vi "Fsweep_SR8XX.vi"() -> ()   [LabVIEW 2020]
panel:
  in  "data acq time (s)":dbl=2.0
  in  "coupled device":enum16{"SRS 8XXX", "Keithley 6221"}(ring)
  in  "base delay (ms)":dbl=2000.0
  in  "test mode":bool=TRUE
  out "done":u32=1
  out "delays (ms)":dbl[](array[numeric])=[4439.024390243903, 4404.322127575027, 4370.113606190229, 4336.391801174221, 4303.149787561701, 4270.38073891527, 4238.07792592359, 4206.234715019476, 4174.844567017659, 4143.901035771921, 4113.3977668513535, 4083.328496235426, 4053.687049027639, 4024.467338187478, 3995.663363280398, 3967.269209245602, 3939.2790451813516, 3911.687123147558, 3884.4877769854065, 3857.675421153779, 3831.244549582238, 3805.189734540312, 3779.505625522889, 3754.1869481514573, 3729.22850309098, 3704.6251649821834, 3680.3718813890364, 3656.4636717612, 3632.895626411248, 3609.6629055064286, 3586.760738074784, 3564.1844210253985, 3541.9293181825924, 3519.990859333863, 3498.364539291357, 3477.045916966707, 3456.0306144590327, 3435.314316155911, 3414.892767847138, 3394.7617758511064, 3374.9172061536083, 3355.354983558889, 3336.071090852786, 3317.0615679777693, 3298.3225112197197, 3279.8500724062824, 3261.640458116619, 3243.6899289024086, 3225.9947985199315, 3208.551433173076, 3191.3562507671204, 3174.4057201731257, 3157.696360502801, 3141.2247403936835, 3124.987477304485, 3108.981236820472, 3093.202731968722, 3077.648722543126, 3062.3160144389926, 3047.2014589971222, 3032.3019523572093, 3017.6144348204493, 3003.135890221209, 2988.863345307645, 2974.793869131124, 2960.924572444339, 2947.2526071079833, 2933.775165505871, 2920.4894799683775, 2907.3928222040795, 2894.482502739488, 2881.755870366748, 2869.2103115991986, 2856.843250134678, 2844.652146326465, 2832.634496661748, 2820.7878332475157, 2809.1097233037576, 2797.597768663886, 2786.24960528225, 2775.0629027486693, 2764.0353638098745, 2753.1647238977457, 2742.448750664277, 2731.8852435231465, 2721.4720331978187, 2711.206981276064, 2701.0879797708303, 2691.112950687351, 2681.279845596418, 2671.5866452137298, 2662.031358985212, 2652.6120246782516, 2643.3267079787383, 2634.173502093844, 2625.1505273604503, 2616.2559308591503, 2607.4878860337403, 2598.8445923161253, 2590.3242747565655, 2581.9251836591748, 2573.645594222615, 2565.483806185897, 2557.43814347922, 2549.506953879787, 2541.6886086725035, 2533.981502315518, 2526.3840521105117, 2518.8946978776826, 2511.5119016353547, 2504.2341472841445, 2497.0599402956186, 2489.9878074053895, 2483.0162963105668, 2476.143975371521, 2469.3694333178873, 2462.691278958754, 2456.108140896974, 2449.618667247538, 2443.2215253599597, 2436.9154015446074, 2430.6990008029316, 2424.571046561526, 2418.5302804099815, 2412.575461842458, 2406.705368002946, 2400.918793434141, 2395.2145498298987, 2389.5914657912076, 2384.048386585637, 2378.5841739102075, 2373.1977056576297, 2367.887875685877, 2362.6535935910315, 2357.493784483362, 2352.4073887665927, 2347.3933619203062, 2342.4506742854455, 2337.578310852868, 2332.7752710549103, 2328.04056855991, 2323.3732310696623, 2318.772300119751, 2314.2368308827204, 2309.7658919740543, 2305.358565260906, 2301.013945673557, 2296.731141019556, 2292.5092718005008, 2288.3474710314285, 2284.2448840627767, 2280.200668404874, 2276.2139935549317, 2272.284040826495, 2268.4100031813205, 2264.591085063646, 2260.82650223682, 2257.1154816222534, 2253.457261140662, 2249.851089555573, 2246.2962263190493, 2242.791941419618, 2239.3375152323556, 2235.932238371111, 2232.5754115428267, 2229.266345403937, 2226.0043604188077, 2222.7887867201857, 2219.6189639716436, 2216.4942412319715, 2213.4139768215036, 2210.3775381903474, 2207.384301788483, 2204.433652937716, 2201.524985705449, 2198.6577027802496, 2195.8312153491884, 2193.044942976925, 2190.298313486511, 2187.590762841889, 2184.9217350320673, 2182.290681956938, 2179.6970633147207, 2177.1403464910118, 2174.620006449405, 2172.1355256236757, 2169.686393811492, 2167.272108069646, 2164.892172610768, 2162.546098701516, 2160.23340456221, 2157.953615267897, 2155.706262650822, 2153.4908852042854, 2151.3070279878743, 2149.154242534032, 2147.032086755969, 2144.940124856872, 2142.8779272404145, 2140.845070422535]
  in  "back to initial frequencies":bool=TRUE
  out "delay sum (min)":dbl=9.36111299636738
  in  "index offset":u16=6
  out "freq profile":dbl[][](array[numeric])=[[40.99999999999999], [41.59176461968469], [42.19207034583551], [42.80104045466266], [43.41880000165687], [44.04547584727021], [44.68119668296755], [45.32609305765421], [45.980297404484844], [46.643944068059355], [47.31716933201128], [48.000111446994545], [48.692910659073924], [49.39570923852533], [50.108651509051946], [50.83188387742187], [51.56555486353358], [52.30981513091526], [53.06481751766459], [53.830717067834826], [54.607671063273884], [55.395839055923275], [56.19538290058288], [57.006466788148714], [57.829257279330584], [58.66392333885625], [59.51063637016918], [60.369570250627405], [61.24090136721011], [62.124808652739766], [63.02147362262691], [63.931080412145505], [64.85381581424615], [65.78986931791488], [66.73943314708613], [67.7027023001168], [68.67987458983036], [69.67115068413874], [70.67673414725078], [71.6968314814753], [72.73165216962732], [73.7814087180468], [74.84631670023795], [75.92659480113835], [77.02246486202736], [78.1341519260824], [79.26188428459274], [80.40589352384065], [81.56641457265877], [82.74368575067426], [83.93794881724882], [85.14944902112572], [86.37843515079277], [87.62515958557246], [88.8898783474497], [90.17285115364719], [91.47434146995997], [92.79461656485945], [94.13394756437879], [95.49260950778984], [96.87088140408437], [98.26904628926995], [99.6873912844931], [101.12620765500114], [102.5857908699552], [104.06644066310672], [105.56846109434923], [107.09216061215888], [108.6378521169361], [110.20585302526148], [111.79648533507905], [113.41007569182058], [115.04695545548357], [116.70746076867859], [118.39193262565769], [120.10071694233959], [121.8341646273455], [123.59263165406033], [125.37647913373338], [127.18607338963533], [129.02178603228427], [130.88399403575826], [132.7730798151091], [134.6894313048933], [136.63344203883705], [138.6055112306498], [140.6060438560061], [142.635450735709], [144.69414862005462], [146.78256027441444], [148.90111456605186], [151.05024655219347], [153.23039756937], [155.44201532404736], [157.68555398456584], [159.961474274406], [162.270243566801], [164.61233598071445], [166.9882324782033], [169.3984209631858], [171.8433963816362], [174.32366082322412], [176.83972362442165], [179.3921014730987], [181.98131851462713], [184.60790645951803], [187.2724046926108], [189.9753603838391], [192.71732860059532], [195.4988724217168], [198.32056305311735], [201.18297994508785], [204.08671091128878], [207.03235224946238], [210.02050886388508], [213.05179438958805], [216.1268313183711], [219.24625112663387], [222.4106944050545], [225.6208109901378], [228.87726009766294], [232.18071045805726], [235.53184045372393], [238.9313382583516], [242.37990197823493], [245.87823979563404], [249.42707011420487], [253.0271217065268], [256.67913386376034], [260.3838565474651], [264.14205054360764], [267.95448761879476], [271.8219506787592], [275.745233929134], [279.7251430385472], [283.7624953040704], [287.85811981905556], [292.01285764339394], [296.22756197623283], [300.50309833118376], [304.84034471406244], [309.2401918031909], [313.703543132304], [318.23131527609524], [322.82443803843955], [327.4838546433357], [332.2105219286013], [337.0054105423655], [341.86950514239686], [346.80380459830866], [351.80932219668233], [356.8870858491522], [362.0381383034912], [367.2635373577478], [372.5643560774688], [377.94168301606044], [383.3966224383289], [388.93029454724626], [394.54383571399273], [400.2383987113154], [406.0151529502572], [411.8752847203018], [417.81999743298553], [423.85051186902433], [429.9680664290081], [436.17391738771397], [442.46933915208774], [448.8556245229529], [455.33408496049384], [461.90605085357], [468.5728717929217], [475.33591684831447], [482.1965748496856], [489.1562546723486], [496.21638552631373], [503.37841724978426], [510.64382060688916], [518.0140875897129], [525.4907317246851], [533.0752883833896], [540.7693150978654], [548.5743918804517], [556.4921215482547], [564.5241300522919], [572.672066811395], [580.937605050924], [589.3224421463751], [597.828299971946], [606.4569252541323], [615.2100899304289], [624.0895915132061], [633.0972534588399], [642.2349255421697], [651.5044842363571], [660.9078330982352], [670.4469031592117], [680.1236533218164], [689.940070761976], [699.8981713370904], [710.0000000000003]]
  out "freqs":dbl[](array[numeric])=[710.0000000000003]
  out "delay (ms)":dbl=2140.845070422535
  out "elapsed time (min)":dbl
  in  "sweep mode":T1(ring)=enum."log"
  in  "size":u32=200
  in  "final":dbl=15000.0
  in  "initial":dbl=41.0
  in  "Device address":refnum<visa-resource-name>[](array[refnum])=["GPIB0::21::INSTR", "GPIB0::22::INSTR", "GPIB0::23::INSTR"]
  # "Test the frequency profile and the estimated measurement time (delay sum (min)) with the 'test mode on'\nTurn the test mode off for the real measurement."
  # "Start data acquistion  and frequency sweeps.\nStop the data acqusition when the sweep is done.\nVISA resource is opened and closed each time a command is executed."
  # "this delay time is added to the frequency dependent delay time"
  # "(1) For multiple lockins, the same freq profile is used but\nbut the starting frequency is offset to prevent crosstalking.\n(2) Ignored for a single lockin. \n* Check the context help"
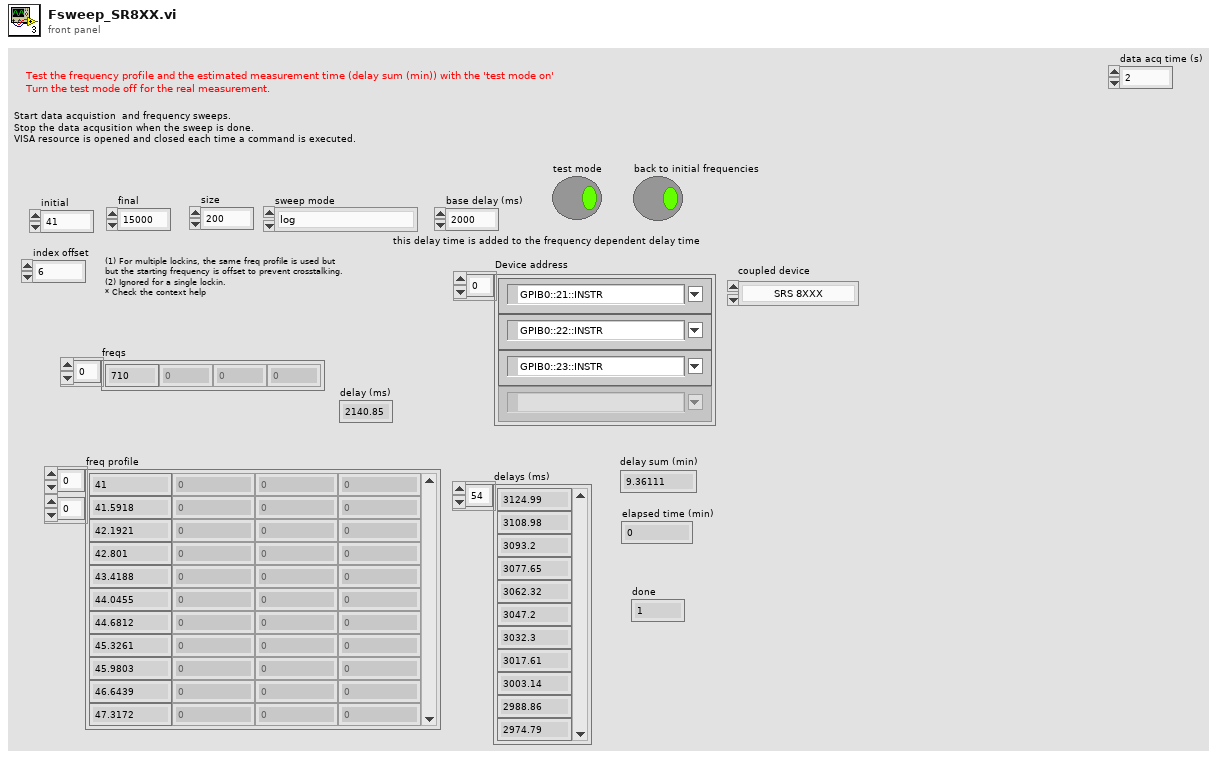
[diagram p1: front panel]
types:
  T1 = enum16{"linear", "inverse", "log", "inverse log"}
  T2 = enum32{"New", "Stop", "Trigger", "Delta Trigger", "Run", "Pause", "comments", "Started?"}
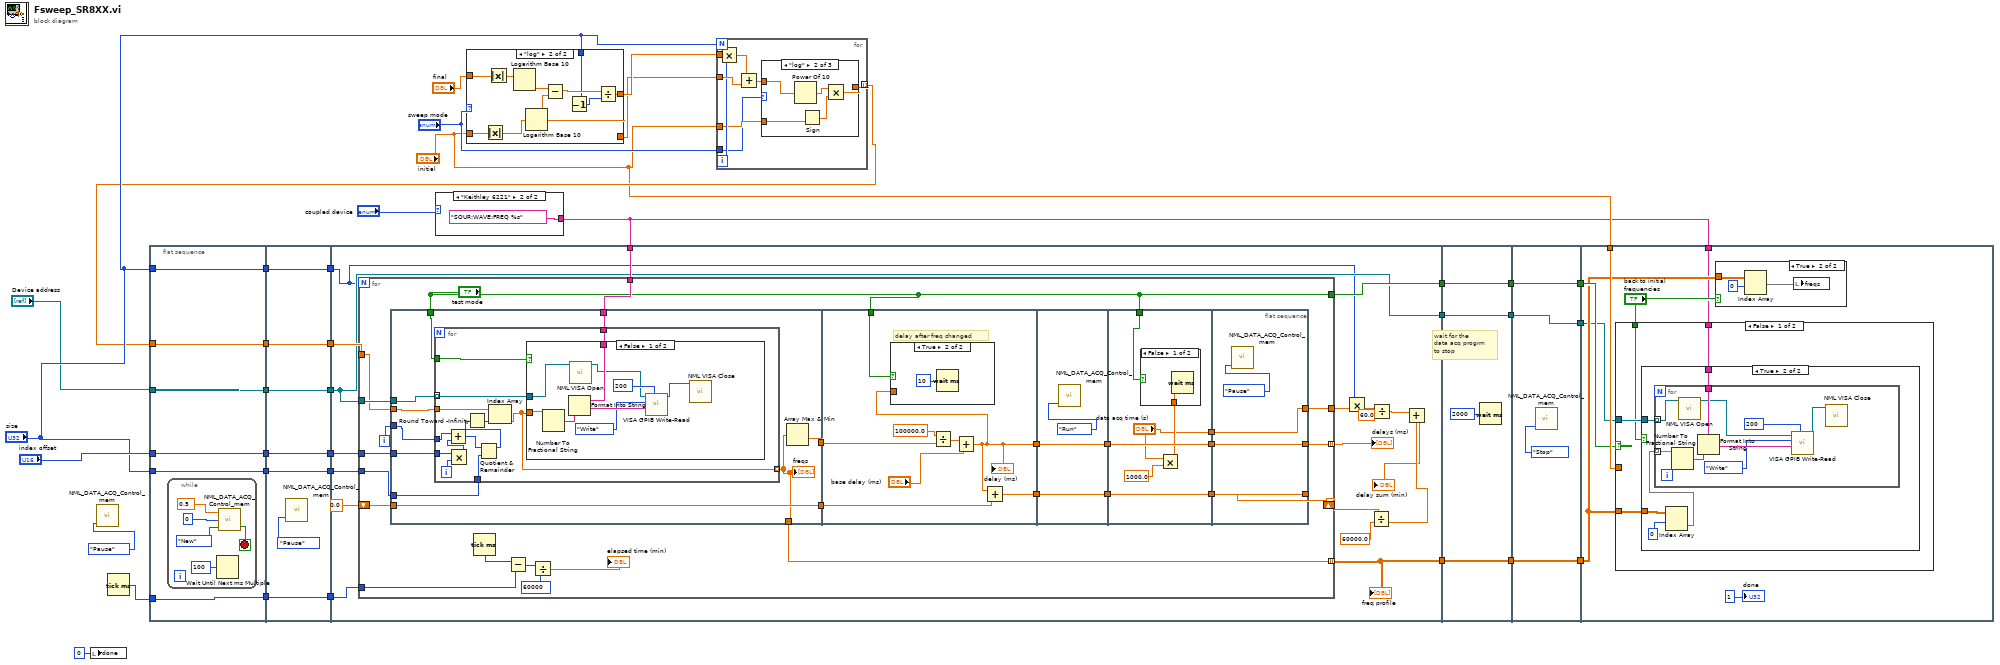
[diagram p0: block diagram]
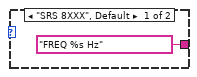
[diagram p2: hidden frame]
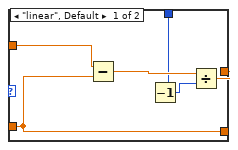
[diagram p3: hidden frame]
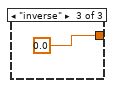
[diagram p5: hidden frame]
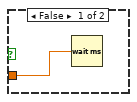
[diagram p7: hidden frame]
diagram:
  n1 = local write "done"(u32 0 ("done")) -> ()
  n2 = call "NML_DATA_ACQ_Control_mem.vi"("Enum"=T2."Pause") -> ()  [unwired: 4 in, 1 out]
  n3 = Tick Count (ms)() -> (millisecond timer value=w35:u32)
  n4 = flat-sequence {
    tunnel: "size" -> [w36]
    tunnel: "index offset" -> [w37]
    tunnel: "Device address" -> [w38]
    tunnel: "size" -> [w39]
    tunnel: w35 -> [w40]
    tunnel: w27 -> [w41]
    tunnel: [w41] -> w19
    tunnel: [w40] -> w17
    tunnel: [w39] -> w15
    tunnel: [w38] -> w13
    tunnel: [w37] -> w11
    tunnel: [w36] -> w9
    tunnel: w19 -> [w53]
    tunnel: [w53] -> w18
    tunnel: w17 -> [w52]
    tunnel: [w52] -> w16
    tunnel: w15 -> [w51]
    tunnel: [w51] -> w14
    tunnel: w13 -> [w50]
    tunnel: [w50] -> w12
    tunnel: w11 -> [w49]
    tunnel: [w49] -> w10
    tunnel: w9 -> [w48]
    tunnel: [w48] -> w8
    tunnel: [w71] -> w6
    tunnel: [w64] -> w4
    tunnel: w22 -> [w62]
    tunnel: [w61] -> w2
    tunnel: w18 -> [w72]
    tunnel: w16 -> [w70]
    tunnel: w14 -> [w59]
    tunnel: w12 -> [w61]
    tunnel: w10 -> [w69]
    tunnel: w8 -> [w68]
    tunnel: w6 -> [w158]
    tunnel: [w158] -> w5
    tunnel: w4 -> [w157]
    tunnel: [w157] -> w3
    tunnel: w2 -> [w156]
    tunnel: [w156] -> w1
    tunnel: w5 -> [w162]
    tunnel: [w162] -> w25
    tunnel: w3 -> [w161]
    tunnel: [w161] -> w24
    tunnel: [w160] -> w21
    tunnel: w1 -> [w160]
    tunnel: w25 -> [w168]
    tunnel: "initial" -> [w169]
    tunnel: w24 -> [w165]
    tunnel: w22 -> [w164]
    tunnel: w21 -> [w163]
    frame #0 {
      n5 = while {
        stop <- w43 stop-if-true
        n6 = Wait Until Next ms Multiple(millisecond multiple=u32 100) -> ()  [unwired: 1 out]
        n7 = call "NML_DATA_ACQ_Control_mem.vi"("Enum"=T2."New", "Trigger Column"=0, "Æ Trigger"=0.5) -> ("started"=w43:bool)  [unwired: 2 in]
      }
    }
    frame #1 {
      n8 = call "NML_DATA_ACQ_Control_mem.vi"("Enum"=T2."Pause") -> ()  [unwired: 4 in, 1 out]
    }
    frame #2 {
      n9 = for {
        N: w59 -> [_]
        tunnel: w72 -> [w83]
        tunnel: ["test mode"] -> w71
        tunnel: w70 -> [w97]
        tunnel: w61 -> [w93]
        tunnel: w69 -> [w91]
        tunnel: w68 -> [w90]
        tunnel: [w84] -> w64 mode=indexing
        tunnel: [w88] -> w63 mode=indexing
        shift-right: [w87] -> w65
        shift-left: 0.0 -> [w85]
        tunnel: w62 -> [w82]
        tunnel: [w73] -> w60
        i -> [w92]
        n10 = flat-sequence {
          tunnel: w83 -> [w106]
          tunnel: "test mode" -> [w108]
          tunnel: w93 -> [w107]
          tunnel: w92 -> [w105]
          tunnel: w91 -> [w104]
          tunnel: w90 -> [w103]
          tunnel: [w101] -> w89
          tunnel: [w100] -> w84
          tunnel: [w102] -> w86
          tunnel: w85 -> [w102]
          tunnel: w82 -> [w99]
          tunnel: w89 -> [w137]
          tunnel: "test mode" -> [w135]
          tunnel: w86 -> [w132]
          tunnel: [w134] -> w81
          tunnel: [w133] -> w80
          tunnel: w81 -> [w143]
          tunnel: w80 -> [w142]
          tunnel: [w143] -> w79
          tunnel: [w142] -> w78
          tunnel: w79 -> [w149]
          tunnel: w78 -> [w148]
          tunnel: [w149] -> w77
          tunnel: [w148] -> w76
          tunnel: "test mode" -> [w145]
          tunnel: ["data acq time (s)"] -> w74
          tunnel: [w153] -> w87
          tunnel: [w154] -> w88
          tunnel: w77 -> [w154]
          tunnel: w76 -> [w153]
          tunnel: w74 -> [w151]
          tunnel: [w151] -> w73
          frame #0 {
            n11 = for {
              tunnel: w108 -> [w121]
              tunnel: w107 -> [w120] mode=indexing
              tunnel: w106 -> [w115]
              tunnel: w105 -> [w118]
              tunnel: w104 -> [w117]
              tunnel: [w112] -> w100 mode=indexing
              tunnel: w103 -> [w113]
              tunnel: w99 -> [w109]
              i -> [w119]
              n12 = Multiply(x=w117, y=w119) -> (x*y=w116:i32)
              n13 = Add(x=w118, y=w116) -> (x+y=w114:i32)
              n14 = Quotient & Remainder(x=w114, y=w113) -> (x-y*floor(x/y)=w111:u32)  [unwired: 1 out]
              n15 = Round Toward -Infinity(1:w111) -> (0:w110:u32)
              n16 = Index Array(array=w115, index=w110) -> (element=w112:dbl)
              n17 = case shown="False" w121 {
                tunnel: w120 -> [w124 _]
                tunnel: w112 -> [w126 _]
                tunnel: w109 -> [w125 _]
                frame False {
                  n18 = Number To Fractional String(number=w126) -> (F-format string=w129:string)  [unwired: 3 in]
                  n19 = Format Into String(format string=w125, w129) -> (resulting string=w130:string)  [unwired: 2 in, 1 out]
                  n20 = call "NML VISA Open.vi"("VISA resource name"=w124) -> ("VISA resource name out"=w123:refnum<visa-resource-name>)  [unwired: 9 in, 1 out]
                  n21 = call "VISA GPIB Write-Read.vi"("Wait (ms)"=u32 200 ("wait (mS)"), "Command"=w130, "Action"=enum16{"Write", "Read", "Write & Read"}."Write", "VISA resource name"=w123) -> ("dup VISA Session"=w122:refnum<visa-resource-name>)  [unwired: 4 in, 3 out]
                  n22 = call "NML VISA Close.vi"("VISA resource name"=w122) -> ()  [unwired: 10 in, 1 out]
                }
                frame True {
                }
              }
            }
            "freqs" <- w100
            n23 = Array Max & Min(array=w100) -> (min value=w101:dbl)  [unwired: 3 out]
          }
          frame #1 {
            # "delay after freq changed"
            n24 = Divide(x=100000.0, y=w137) -> (x/y=w138:dbl)
            n25 = Add(x=w138, y="base delay (ms)") -> (x+y=w134:dbl)
            "delay (ms)" <- w134
            n26 = case shown="True" w135 {
              tunnel: w134 -> [w139 _]
              frame False {
                n27 = Wait (ms)(milliseconds to wait=w139) -> ()  [unwired: 1 out]
              }
              frame True {
                n28 = Wait (ms)(milliseconds to wait=u32 10) -> ()  [unwired: 1 out]
              }
            }
            n29 = Add(x=w134, y=w132) -> (x+y=w133:dbl)
          }
          frame #2 {
            n30 = call "NML_DATA_ACQ_Control_mem.vi"("Enum"=T2."Run") -> ()  [unwired: 4 in, 1 out]
          }
          frame #3 {
            n31 = Multiply(x="data acq time (s)", y=1000.0) -> (x*y=w146:dbl)
            n32 = case shown="False" w145 {
              tunnel: w146 -> [w150 _]
              frame False {
                n33 = Wait (ms)(milliseconds to wait=w150) -> ()  [unwired: 1 out]
              }
              frame True {
              }
            }
          }
          frame #4 {
            n34 = call "NML_DATA_ACQ_Control_mem.vi"("Enum"=T2."Pause") -> ()  [unwired: 4 in, 1 out]
          }
        }
        n35 = Tick Count (ms)() -> (millisecond timer value=w98:u32)
        n36 = Subtract(x=w98, y=w97) -> (x-y=w96:u32)
        n37 = Divide(x=w96, y=u32 60000) -> (x/y=→"elapsed time (min)":dbl)
      }
      "freq profile" <- w64
      "delays (ms)" <- w63
      n38 = Multiply(x=w59, y=w60) -> (x*y=w58:dbl)
      n39 = Divide(x=w65, y=60000.0) -> (x/y=w55:dbl)
      n40 = Divide(x=w58, y=60.0) -> (x/y=w56:dbl)
      n41 = Add(x=w56, y=w55) -> (x+y=→"delay sum (min)":dbl)
    }
    frame #3 {
      # "wait for the\ndata acq progrm\nto stop"
      n42 = Wait (ms)(milliseconds to wait=u32 2000) -> ()  [unwired: 1 out]
    }
    frame #4 {
      n43 = call "NML_DATA_ACQ_Control_mem.vi"("Enum"=T2."Stop") -> ()  [unwired: 4 in, 1 out]
    }
    frame #5 {
      n44 = case shown="False" w168 {
        tunnel: w169 -> [_ _]
        tunnel: w163 -> [w176 _]
        tunnel: w165 -> [w175 _]
        tunnel: "back to initial frequencies" -> [w174 _]
        tunnel: w164 -> [w173 _]
        frame False {
          n45 = case shown="True" w174 {
            tunnel: w176 -> [_ w181]
            tunnel: w175 -> [_ w180]
            tunnel: w173 -> [_ w177]
            frame False {
            }
            frame True {
              n46 = Index Array(array=w180, index (row)=0) -> (element=w178:dbl[])  [unwired: 1 in]
              n47 = for {
                tunnel: w181 -> [w184] mode=indexing
                tunnel: w178 -> [w186] mode=indexing
                tunnel: w177 -> [w185]
                n48 = Number To Fractional String(number=w186) -> (F-format string=w189:string)  [unwired: 3 in]
                n49 = call "NML VISA Open.vi"("VISA resource name"=w184) -> ("VISA resource name out"=w183:refnum<visa-resource-name>)  [unwired: 9 in, 1 out]
                n50 = Format Into String(format string=w185, w189) -> (resulting string=w190:string)  [unwired: 2 in, 1 out]
                n51 = call "VISA GPIB Write-Read.vi"("Wait (ms)"=u32 200 ("wait (mS)"), "Command"=w190, "Action"=enum16{"Write", "Read", "Write & Read"}."Write", "VISA resource name"=w183) -> ("dup VISA Session"=w182:refnum<visa-resource-name>)  [unwired: 4 in, 3 out]
                n52 = call "NML VISA Close.vi"("VISA resource name"=w182) -> ()  [unwired: 10 in, 1 out]
              }
            }
          }
        }
        frame True {
        }
      }
      n53 = case shown="True" "back to initial frequencies" {
        tunnel: w165 -> [_ w172]
        frame False {
        }
        frame True {
          n54 = Index Array(array=w172, index (row)=0) -> (element=w170:dbl[])  [unwired: 1 in]
          n55 = local write "freqs"(w170) -> ()
        }
      }
      "done" <- u32 1 ("done")
    }
  }
  n56 = case shown="\"Keithley 6221\"" "coupled device" {
    tunnel: ["FREQ %s Hz" ("format string") "SOUR:WAVE:FREQ %s" ("format string")] -> w22
    frame "SRS 8XXX", Default {
    }
    frame "Keithley 6221" {
    }
  }
  n57 = case shown="\"log\"" "sweep mode" {
    tunnel: "final" -> [w198 w199]
    tunnel: "initial" -> [w193 w204]
    tunnel: "size" -> [w196 w207]
    tunnel: [w195 w206] -> w32
    tunnel: [w193 w200] -> w31
    frame "linear", Default {
      n58 = Subtract(x=w198, y=w193) -> (x-y=w197:dbl)
      n59 = Decrement(x=w196) -> (x-1=w194:u32)
      n60 = Divide(x=w197, y=w194) -> (x/y=w195:dbl)
    }
    frame "log" {
      n61 = Absolute Value(x=w204) -> (abs(x)=w201:dbl)
      n62 = Absolute Value(x=w199) -> (abs(x)=w202:dbl)
      n63 = Logarithm Base 10(1:w202) -> (0:w203:dbl)
      n64 = Logarithm Base 10(1:w201) -> (0:w200:dbl)
      n65 = Subtract(x=w203, y=w200) -> (x-y=w208:dbl)
      n66 = Decrement(x=w207) -> (x-1=w205:u32)
      n67 = Divide(x=w208, y=w205) -> (x/y=w206:dbl)
    }
  }
  n68 = for {
    N: "size" -> [_]
    tunnel: w32 -> [w214]
    tunnel: [w216] -> w27 mode=indexing
    tunnel: "sweep mode" -> [w209]
    tunnel: w31 -> [w212]
    tunnel: "initial" -> [w210]
    i -> [w211]
    n69 = Multiply(x=w214, y=w211) -> (x*y=w213:dbl)
    n70 = Add(x=w213, y=w212) -> (x+y=w215:dbl)
    n71 = case shown="\"log\"" w209 {
      tunnel: [w217 w220 0.0] -> w216
      tunnel: w215 -> [w217 w222 _]
      tunnel: w210 -> [_ w219 _]
      frame "linear", Default {
      }
      frame "log" {
        n72 = Power Of 10(x=w222) -> (10^x=w221:dbl)
        n73 = Sign(1:w219) -> (0:w218:dbl)
        n74 = Multiply(x=w221, y=w218) -> (x*y=w220:dbl)
      }
      frame "inverse" {
      }
    }
  }
